vi "Shift Rev.vi"(10 "iterator":refnum<data-value>, 11 "Node in":refnum<class "Node.lvclass">) -> (3 "Node out":refnum<class "Node.lvclass">)   [LabVIEW 2021, in "d20.lvlib" / "Node.lvclass"]
uses:
  Node.lvclass
  INode/INode.lvclass
  Node.lvclass/Node.ctl
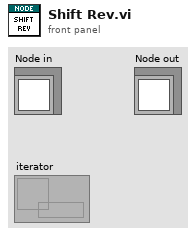
[diagram p1: front panel]
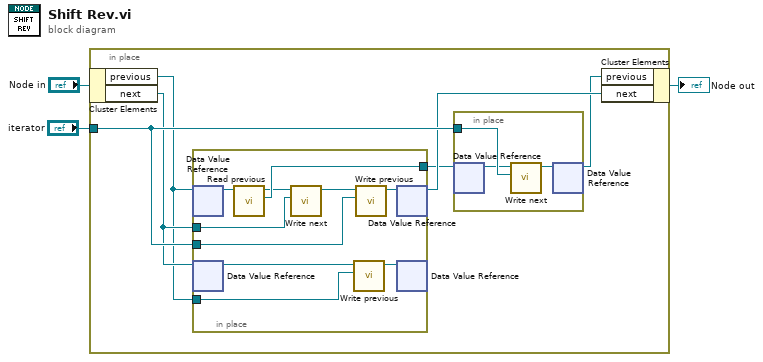
[diagram p0: block diagram]
diagram:
  n1 = in-place {
    in-place-border: "iterator" -> [w9]
    n2 = in-place-cluster #1("Node in") -> ("previous"=w7:refnum<data-value>, "next"=w8:refnum<data-value>)
    n3 = in-place {
      in-place-border: w7 -> [w14]
      in-place-border: [w19] -> w5
      in-place-border: w8 -> [w17]
      in-place-border: w9 -> [w15]
      n4 = in-place-dvr #2(w7) -> (w12:refnum<class "INode.lvclass">)  [unwired: 1 out]
      n5 = in-place-dvr #3(w8) -> (w11:refnum<class "INode.lvclass">)  [unwired: 1 out]
      n6 = call-dynamic "Read previous.vi"("Node in"=w12) -> ("previous"=w19:refnum<data-value>, "Node out"=w18:refnum<class "INode.lvclass">)  [unwired: 9 in]
      n7 = call-dynamic "Write next.vi"("next"=w17, "Node in"=w18) -> ("Node out"=w16:refnum<class "INode.lvclass">)  [unwired: 9 in]
      n8 = call-dynamic "Write previous.vi"("previous"=w14, "Node in"=w11) -> ("Node out"=w10:refnum<class "INode.lvclass">)  [unwired: 9 in]
      n9 = call-dynamic "Write previous.vi"("previous"=w15, "Node in"=w16) -> ("Node out"=w13:refnum<class "INode.lvclass">)  [unwired: 9 in]
      n10 = in-place-dvr #2(w13) -> (w6:refnum<data-value>)  [unwired: 1 out]
      n11 = in-place-dvr #3(w10) -> ()  [unwired: 2 out]
    }
    n12 = in-place {
      in-place-border: w9 -> [w22]
      n13 = in-place-dvr #4(w5) -> (w21:refnum<class "INode.lvclass">)  [unwired: 1 out]
      n14 = call-dynamic "Write next.vi"("next"=w22, "Node in"=w21) -> ("Node out"=w20:refnum<class "INode.lvclass">)  [unwired: 9 in]
      n15 = in-place-dvr #4(w20) -> (w4:refnum<data-value>)  [unwired: 1 out]
    }
    n16 = in-place-cluster #1("previous"=w4, "next"=w6) -> (→"Node out":refnum<class "Node.lvclass">)
  }
